vi "Launch panel asynchronously.vi"(6 "Fiber Auto Collimation state data":refnum<class "Fiber Auto Collimation state data.lvclass">, 7 "Station config":refnum<class "Station config.lvclass">, 8 "error in":errorcluster, 9 "Start hidden? (F)":bool, 10 "Clone name (blank = only one instance)":string, 11 "Fiber Auto Collimation panel in":refnum<class "Fiber Auto Collimation panel.lvclass">) -> (0 "error out":errorcluster, 3 "Fiber Auto Collimation panel out":refnum<class "Fiber Auto Collimation panel.lvclass">)   [LabVIEW 2018, in "Fiber Auto Collimation panel.lvclass"]
doc: "This VI launches the panel associated with its class, then returns after the panel was launched successfully and asynchronously. The return value will contain the clone name and a reference to the VI of the launched panel, if successful.\n\nIf the class launching this panel supports multiple instances of its panel at once, the \"Clone name\" input cannot be blank and will generate an error when called.\n\nIf this is called on the top-level class, an error is generated as it does not have a launchable panel (it's the default Main VI).\n\nThe station config and state data inputs are meant mostly to be initial seeds for a panel as it perform its initial setup. Neither should be altered in this VI, which is why there is no output for those wires.\n\n\"Start hidden\", if True, instructs the panel to not show itself when it's done loading and registering for events. This should be selected if the panel in question either will be immediately placed into a sub-panel or if it will wait to self-reveal itself later due to a change in state data."
uses:
  Fiber Auto Collimation panel.lvclass
  State data/Fiber Auto Collimation state data.lvclass
  <userlib>/Recipe/Station Config/Station config.lvclass
  Fiber Auto Collimation panel.lvclass/Fiber Auto Collimation panel.ctl
  c14db125-76c7-4d61-b482-ed49ef3dce96.vi
  <vilib>/Utility/error.llb/Clear Errors.vi
  <userlib>/nLight Error Handling/Log any errors.vi
  <vilib>/Utility/LVClass/Get LV Class Name.vi
  <userlib>/nLight Error Handling/Merge errors no loss.vi
  References/Fiber Auto Collimation References.lvclass
panel:
  out "Numeric":i32
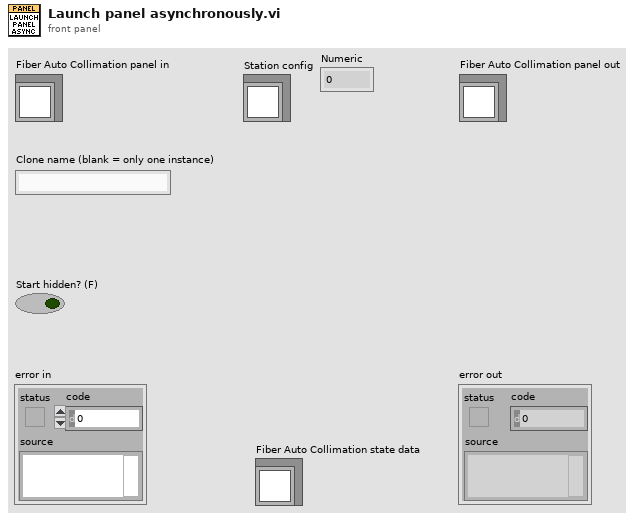
[diagram p1: front panel]
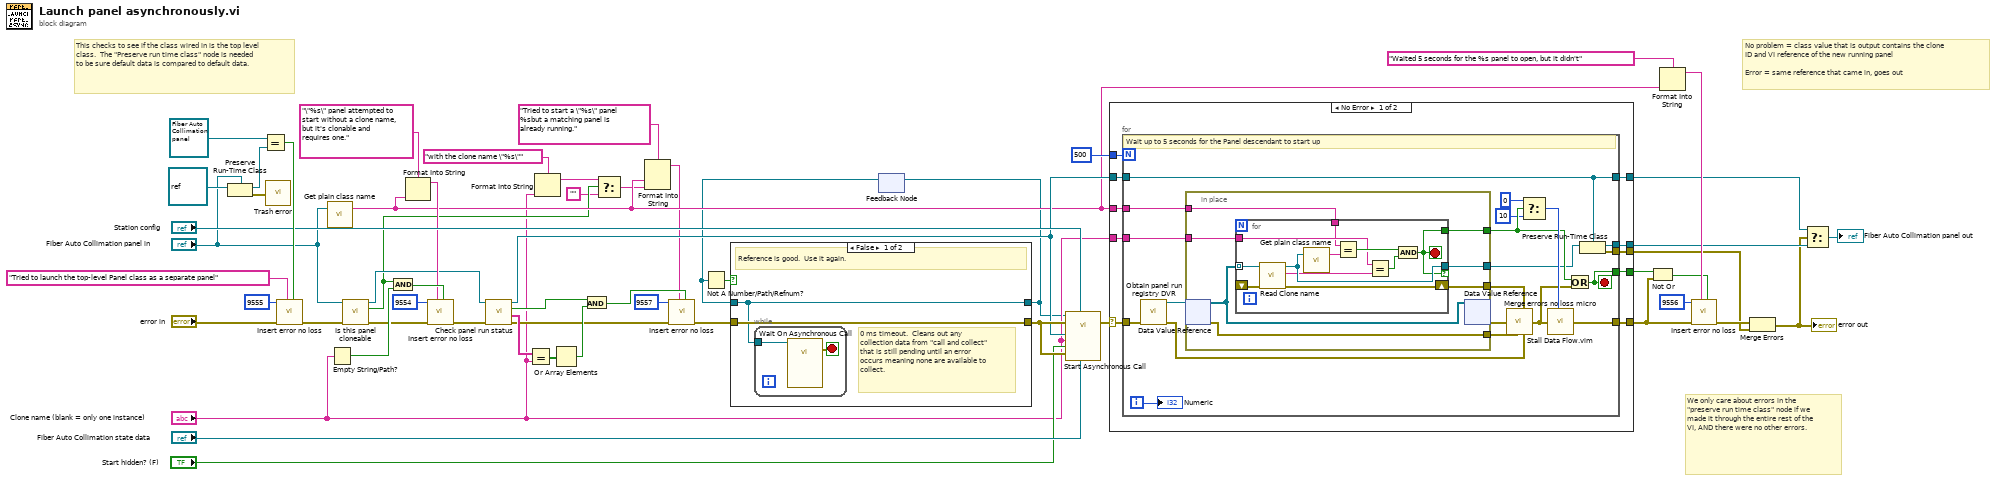
[diagram p0: block diagram]
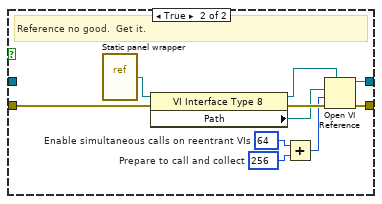
[diagram p2: hidden frame]
diagram:
  # "We only care about errors in the \"preserve run time class\" node if we made it through the entire rest of the VI, AND there were no other errors."
  # "No problem = class value that is output contains the clone ID and VI reference of the new running panel\n\nError = same reference that came in, goes out"
  # "This checks to see if the class wired in is the top level class.  The \"Preserve run time class\" node is needed to be sure default data is compared to default data."
  n1 = Preserve Run-Time Class(object in=refnum<class> refnum ("LabVIEW Object"), 2:"Fiber Auto Collimation panel in") -> (object out=w55:refnum<class "Fiber Auto Collimation panel.lvclass">, error out=w30:errorcluster)  [unwired: 1 in]
  n2 = Equal?(x=refnum<class "Fiber Auto Collimation panel.lvclass"> refnum ("nLight Station Template panel in"), y=w55) -> (x = y?=w53:bool)
  n3 = call <userlib>:"Trash error.vi"("error in"=w30) -> ()  [unwired: 15 in]
  n4 = call <userlib>:"Insert error no loss.vi"("Add error? (T)"=w53, "error message"="Tried to launch the top-level Panel class as a separate panel", "error in (no error)"="error in", "error code"=9555) -> ("error out"=w38:errorcluster)  [unwired: 5 in]
  n5 = call <userlib>:"Get plain class name.vi"("Any class"="Fiber Auto Collimation panel in") -> ("Plain class name"=w11:string)  [unwired: 2 in]
  n6 = Empty String/Path?(string/path="Clone name (blank = only one instance)") -> (empty?=w37:bool)
  n7 = call-dynamic "Is this panel cloneable.vi"("error in (no error)"=w38, "Fiber Auto Collimation panel in"="Fiber Auto Collimation panel in") -> ("error out"=w34:errorcluster, "This class is cloneable"=w9:bool, "Fiber Auto Collimation panel out"=w22:refnum<class "Fiber Auto Collimation panel.lvclass">)  [unwired: 7 in]
  n8 = And(x=w9, y=w37) -> (x .and. y?=w35:bool)
  n9 = Format Into String(format string="\"%s\" panel attempted to start without a clone name, but it's clonable and requires one.", w11) -> (resulting string=w31:string)  [unwired: 2 in, 1 out]
  n10 = call <userlib>:"Insert error no loss.vi"("Add error? (T)"=w35, "error message"=w31, "error in (no error)"=w34, "error code"=9554) -> ("error out"=w23:errorcluster)  [unwired: 5 in]
  n11 = call "Check panel run status.vi"("error in (no error)"=w23, "Fiber Auto Collimation panel in"=w22) -> ("error out"=w15:errorcluster, "Clone names running"=w19:string[], "Panel(s) running"=w20:bool, "Fiber Auto Collimation panel out"=w21:refnum<class "Fiber Auto Collimation panel.lvclass">)  [unwired: 6 in]
  n12 = Equal?(x=w19, y="Clone name (blank = only one instance)") -> (x = y?=w18:bool[])
  n13 = Format Into String(format string="with the clone name \"%s\"", "Clone name (blank = only one instance)") -> (resulting string=w7:string)  [unwired: 2 in, 1 out]
  n14 = Or Array Elements(Boolean array=w18) -> (logical OR=w17:bool)
  n15 = And(x=w20, y=w17) -> (x .and. y?=w13:bool)
  n16 = Select(t=w7, s=w9, f="") -> (s? t:f=w4:string)
  n17 = Format Into String(format string="Tried to start a \"%s\" panel %sbut a matching panel is already running.", w11, w4) -> (resulting string=w10:string)  [unwired: 2 in, 1 out]
  n18 = call <userlib>:"Insert error no loss.vi"("Add error? (T)"=w13, "error message"=w10, "error in (no error)"=w15, "error code"=9557) -> ("error out"=w14:errorcluster)  [unwired: 5 in]
  n19 = feedback #1() -> (w1:refnum<vi>)  [unwired: 1 in]
  n20 = Not A Number/Path/Refnum?(number/path/refnum=w1) -> (NaN/Path/Refnum?=w2:bool)
  n21 = case shown="False" w2 {
    tunnel: [w58 w64] -> w3
    tunnel: [w59 w63] -> w28
    tunnel: w14 -> [w59 w62]
    tunnel: w1 -> [w58 _]
    frame False {
      # "0 ms timeout.  Cleans out any collection data from \"call and collect\" that is still pending until an error occurs meaning none are available to collect."
      # "Reference is good.  Use it again."
      n22 = while {
        tunnel: w58 -> [w61]
        stop <- w60 stop-if-true
        n23 = call-by-ref "Wait On Asynchronous Call"(reference=w61) -> (error out=w60:errorcluster)  [unwired: 11 in, 3 out]
      }
    }
    frame True {
      w66 = 256  # Prepare to call and collect
      w67 = 64  # Enable simultaneous calls on reentrant VIs
      # "Reference no good.  Get it."
      n24 = vi-ref "Static panel wrapper.vi"() -> (w71:refnum<vi>)
      n25 = property class="VI Interface Type 8"(reference=w71, error in=w62) -> (reference out=w68:refnum<vi>, error out=w70:errorcluster, "Path"=w69:path)
      n26 = Add(x=w67, y=w66) -> (x+y=w65:i32)
      n27 = Open VI Reference(type specifier VI Refnum (for type only)=w68, vi path=w69, options=w65, error in (no error)=w70) -> (vi reference=w64:refnum<vi>, error out=w63:errorcluster)  [unwired: 2 in]
    }
  }
  n28 = feedback-in #1(w3) -> ()
  n29 = call-by-ref "Start Asynchronous Call"(reference=w3, error in=w28, "Fiber Auto Collimation state data"="Fiber Auto Collimation state data", "Station config"="Station config", 8:"error in (no error)"=w28, "Start hidden?"="Start hidden? (F)", "Clone name [blank = only one instance]"="Clone name (blank = only one instance)", "nLight Station Template panel in"=w21) -> (error out=w48:errorcluster)  [unwired: 4 in, 3 out]
  n30 = case shown="No Error" w48 {
    selector: w48 -> [w80 w121]
    tunnel: 500 -> [w81 _]
    tunnel: [w79 w121] -> w47
    tunnel: [w78 _] -> w46
    tunnel: [w77 w120] -> w41
    tunnel: [w76 w120] -> w39
    tunnel: w21 -> [w75 w120]
    tunnel: "Clone name (blank = only one instance)" -> [w74 _]
    tunnel: w11 -> [w73 _]
    tunnel: [w72 _] -> w25
    frame No Error {
      n31 = for {
        N: w81 -> [_]
        tunnel: w75 -> [w88]
        tunnel: w74 -> [w99]
        tunnel: [w90] -> w77
        tunnel: [w85] -> w78
        tunnel: w73 -> [w89]
        tunnel: [w88] -> w76
        tunnel: w80 -> [w100]
        tunnel: [w83] -> w79
        tunnel: [w82] -> w72
        i -> [w87]
        stop <- w85 stop-if-true
        # "Wait up to 5 seconds for the Panel descendant to start up"
        n32 = call "Obtain panel run registry DVR.vi"("error in"=w100) -> ("error out"=w94:errorcluster, "Panel registration DVR"=w101:refnum<data-value>)  [unwired: 9 in]
        n33 = in-place {
          in-place-border: [w108] -> w95
          in-place-border: [w107] -> w93
          in-place-border: [w105] -> w91
          in-place-border: w99 -> [w104]
          in-place-border: [w103] -> w92
          in-place-border: w89 -> [w102]
          n34 = in-place-dvr #2(w101) -> (w106:refnum<class "Fiber Auto Collimation panel.lvclass">[], w108:errorcluster)
          n35 = for {
            tunnel: w106 -> [w119] mode=indexing
            shift-right: [w117] -> w107
            shift-left: _ -> [w118]
            tunnel: [w114] -> w105 if=w110
            tunnel: w104 -> [w112]
            tunnel: [w110] -> w103
            tunnel: w102 -> [w109]
            stop <- w110 stop-if-true
            n36 = call "Read Clone name.vi"("error in (no error)"=w118, "Fiber Auto Collimation panel in"=w119) -> ("error out"=w117:errorcluster, "Clone name"=w113:string, "Fiber Auto Collimation panel out"=w114:refnum<class "Fiber Auto Collimation panel.lvclass">)  [unwired: 7 in]
            n37 = call <userlib>:"Get plain class name.vi"("Any class"=w114) -> ("Plain class name"=w116:string)  [unwired: 2 in]
            n38 = Equal?(x=w109, y=w116) -> (x = y?=w115:bool)
            n39 = Equal?(x=w112, y=w113) -> (x = y?=w111:bool)
            n40 = And(x=w115, y=w111) -> (x .and. y?=w110:bool)
          }
          n41 = in-place-dvr #2(w106) -> (w96:errorcluster)  [unwired: 1 out]
        }
        n42 = call <userlib>:"Merge errors no loss micro.vi"("error in (no error) 1"=w96, "error in (no error) 5"=w95, "error in (no error) 3"=w93, "error in (no error) 6"=w94) -> ("error out"=w86:errorcluster)  [unwired: 5 in]
        n43 = Select(t=u32 0 ("milliseconds to wait"), s=w92, f=u32 10 ("milliseconds to wait")) -> (s? t:f=w97:u32)
        n44 = call "Stall Data Flow.vim"("value in"=w86, "milliseconds to wait"=w97) -> ("value out"=w83:errorcluster)  [unwired: 1 out]
        n45 = Or(x=w92, y=w86) -> (x .or. y?=w85:bool)
        n46 = Preserve Run-Time Class(object in=w91, 2:w88) -> (object out=w90:refnum<class "Fiber Auto Collimation panel.lvclass">, error out=w82:errorcluster)  [unwired: 1 in]
        "Numeric" <- w87
      }
    }
    frame Error {
    }
  }
  n47 = Not Or(1:w47, 2:w46) -> (0:w42:bool)
  n48 = Format Into String(format string="Waited 5 seconds for the %s panel to open, but it didn't", w11) -> (resulting string=w43:string)  [unwired: 2 in, 1 out]
  n49 = call <userlib>:"Insert error no loss.vi"("Add error? (T)"=w42, "error message"=w43, "error in (no error)"=w47, "error code"=9556) -> ("error out"=w27:errorcluster)  [unwired: 5 in]
  n50 = Merge Errors(w27, w25) -> (w26:errorcluster)
  "error out" <- w26
  n51 = Select(t=w39, s=w26, f=w41) -> (s? t:f=→"Fiber Auto Collimation panel out":refnum<class "Fiber Auto Collimation panel.lvclass">)
